vi "Decide Action.vi"(8 "error in (no error)":errorcluster, 11 "Mouse in":refnum<class "Mouse.lvclass">) -> (0 "error out":errorcluster, 2 "Action":T1, 3 "Mouse out":refnum<class "Mouse.lvclass">)   [LabVIEW 2020, in "Maze.lvlib" / "Mouse.lvclass"]
doc: "This is the only VI that is 100% necessary to implement for the mouse algorithm (besides the Author property). This VI is called each step of the run to allow the mouse to decide what action it will take which is either: <b>Turn Left</b>, <b>Turn Right</b>, or <b>Move Forward</b>.\n\nIf a mouse runs headfirst into a wall (remember your step speed is merely the simulation speed and not indicative of the speeds at which racing mice are capable of making decisions and running at) its run will be stopped and <i>Crash.vi</i> will be called so the mouse knows it has crashed and the run is ending."
uses:
  Mouse.lvclass
  Action.ctl
  Maze.lvlib
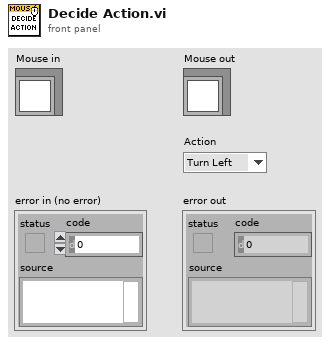
[diagram p1: front panel]
types:
  T1 = typedef "Maze.lvlib/Action.ctl" = enum16{"Turn Left", "Turn Right", "Forward"}
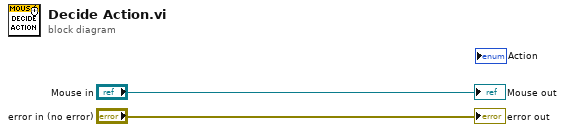
[diagram p0: block diagram]
diagram:
  "error out" <- "error in (no error)"
  "Mouse out" <- "Mouse in"
